vi "Publish to Subscribers.vi"(8 "error in (no error)":errorcluster, 10 "Message Data":variant, 11 "Domino Laser module Class in":refnum<class "Domino Laser module Class.lvclass">) -> (0 "error out":errorcluster, 3 "Domino Laser module Class out":refnum<class "Domino Laser module Class.lvclass">)   [LabVIEW 2024, in "Domino LM.lvlib" / "Domino Laser module Class.lvclass"]
uses:
  CTRLS/Domino Laser module Class.lvclass
  CTRLS/Domino Laser module Class.lvclass/Domino Laser module Class.ctl
  ARCH/Message Queue/Message Cluster.ctl
  ARCH/Message Queue/Message Queue.lvlib
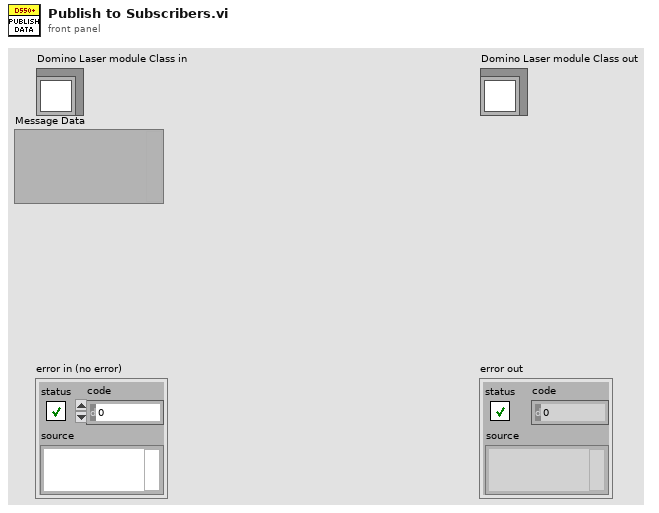
[diagram p1: front panel]
types:
  T1 = typedef "Message Queue.lvlib/Message Cluster.ctl" = cluster{"Message":string, "Message Data":variant}
  T2 = cluster{"Subscriber Message":string, "Subscribe Queue":refnum<queue>}[]
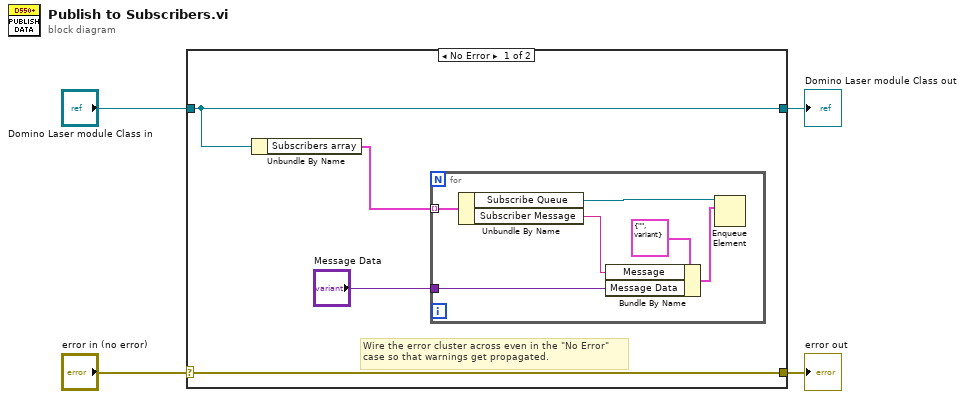
[diagram p0: block diagram]
diagram:
  n1 = case shown="No Error" "error in (no error)" {
    selector: "error in (no error)" -> [w8 w16]
    tunnel: [w8 w16] -> w3
    tunnel: [w6 w15] -> w1
    tunnel: "Domino Laser module Class in" -> [w6 w15]
    frame No Error {
      # "Wire the error cluster across even in the \"No Error\"\ncase so that warnings get propagated."
      n2 = Unbundle By Name(w6) -> ("Subscribers array"=w7:T2)
      n3 = for {
        tunnel: w7 -> [w14] mode=indexing
        tunnel: "Message Data" -> [w9]
        n4 = Unbundle By Name(w14) -> ("Subscribe Queue"=w13:refnum<queue>, "Subscriber Message"=w10:string)
        n5 = Bundle By Name(cluster=T1 {"Message"="", "Message Data"=variant} ("element"), "Message"=w10, "Message Data"=w9) -> (w11:T1)
        n6 = Enqueue Element(queue=w13, element=w11) -> ()  [unwired: 2 in, 3 out]
      }
    }
    frame Error {
    }
  }
  "error out" <- w3
  "Domino Laser module Class out" <- w1
